vi "Add(DBL).vi"(1 "Enable(T)":bool=TRUE, 2 "In":dbl, 4 "n":dbl=1.0) -> (6 "Out":dbl=1.0 format="%.2f")   [LabVIEW 2013]
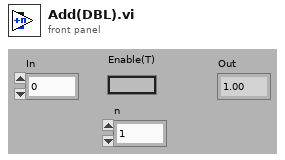
[diagram p1: front panel]
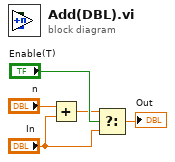
[diagram p0: block diagram]
diagram:
  n1 = Add(x="n", y="In") -> (x+y=w1:dbl)
  n2 = Select(t=w1, s="Enable(T)", f="In") -> (s? t:f=→"Out":dbl)
